vi "eWriteNames and eReadNames.vi"(0 "Handle In":i32, 1 "aReadNames":string[](array[string]), 5 "aWriteNames":string[](array[string]), 9 "aWriteValues":dbl[](array[numeric]) format="%.2f", 11 "error in":errorcluster) -> (4 "Handle Out":i32, 10 "aReadValues":dbl[](array[numeric]) format="%.2f", 15 "error out":errorcluster)   [LabVIEW 2024]
panel:
  out "Error String":string
  # "The VIs in the \\Functions folder are the basic function calls from the LJM library and\nare set up as sub-VIs that need to be called by some parent VI.  Those LJM functions\ncan do everything including combined writes and reads in a single packet.\n\nThis utility VI does 2 LJM calls ... a call to eReadNames followed by a call to\neWriteNames ... which will result in at least 2 low-level modbus transactions.  This can\nbe done more efficiently with eNames which will use 1 modbus transaction if\npossible, but this utility VI might be a simpler option when max speed is not important."
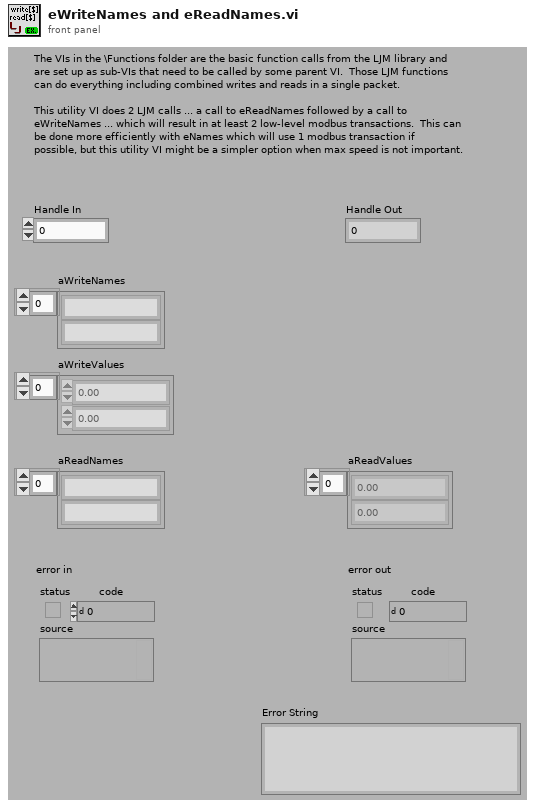
[diagram p1: front panel]
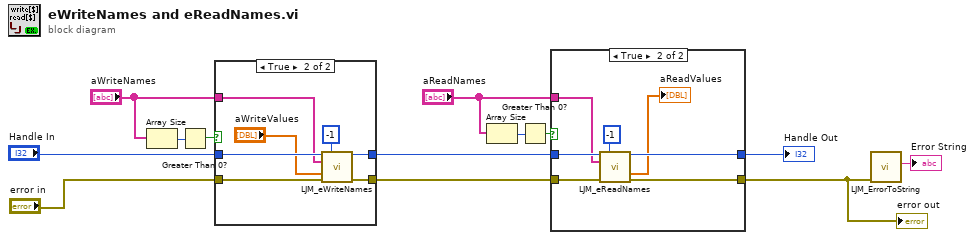
[diagram p0: block diagram]
diagram:
  n1 = Array Size(array="aWriteNames") -> (size(s)=w5:i32)
  n2 = Greater Than 0?(x=w5) -> (x > 0?=w6:bool)
  n3 = case shown="True" w6 {
    tunnel: "Handle In" -> [w15 w22]
    tunnel: "error in" -> [w14 w21]
    tunnel: [w14 w20] -> w10
    tunnel: [w15 w19] -> w9
    tunnel: "aWriteNames" -> [_ w18]
    frame False {
    }
    frame True {
      n4 = call "LJM_eWriteNames.vi"("Handle In"=w22, "NumFrames (Auto-Detect)"=-1, "aNames"=w18, "aValuesIn"="aWriteValues", "error in"=w21) -> ("Handle Out"=w19:i32, "error out"=w20:errorcluster)  [unwired: 8 in, 1 out]
    }
  }
  n5 = Array Size(array="aReadNames") -> (size(s)=w3:i32)
  n6 = Greater Than 0?(x=w3) -> (x > 0?=w1:bool)
  n7 = case shown="True" w1 {
    tunnel: w10 -> [w23 w31]
    tunnel: w9 -> [w24 w30]
    tunnel: [w24 w29] -> w8
    tunnel: [w23 w28] -> w7
    tunnel: "aReadNames" -> [_ w27]
    frame False {
    }
    frame True {
      n8 = call "LJM_eReadNames.vi"("Handle In"=w30, "NumFrames (Auto-Detect)"=-1, "aNames"=w27, "error in"=w31) -> ("Handle Out"=w29:i32, "aValuesOut"=→"aReadValues":dbl[], "error out"=w28:errorcluster)  [unwired: 8 in, 1 out]
    }
  }
  "error out" <- w7
  "Handle Out" <- w8
  n9 = call "LJM_ErrorToString.vi"("error in"=w7) -> ("String"=→"Error String":string)  [unwired: 10 in]
